vi "Teardown.vi"(8 "error in (no error)":errorcluster, 11 "Test Case Test Double In":refnum<class "Test Case Test Double.lvclass">) -> (0 "error out":errorcluster, 3 "Test Case Test Double Out":refnum<class "Test Case Test Double.lvclass">)   [LabVIEW 2020, in "Test Case Test Double.lvclass"]
uses:
  Test Case Test Double.lvclass
  source/Framework/Test Case/LUnit Test Case.lvclass
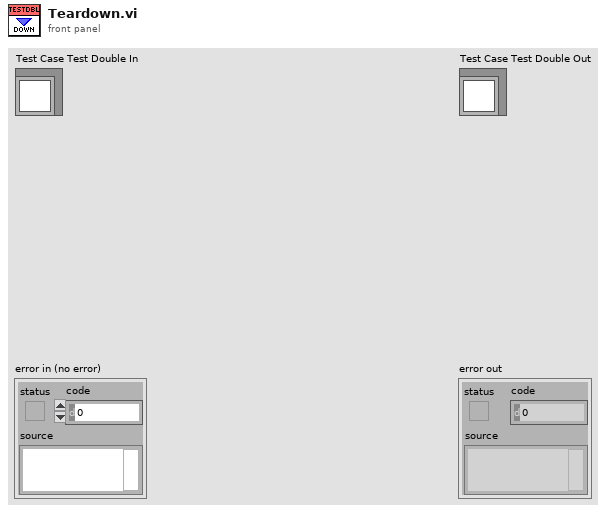
[diagram p1: front panel]
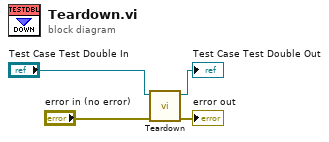
[diagram p0: block diagram]
diagram:
  n1 = call-parent "Teardown.vi"("error in (no error)"="error in (no error)", "LUnit Test Case In"="Test Case Test Double In") -> ("error out"=→"error out":errorcluster, "LUnit Test Case Out"=→"Test Case Test Double Out":refnum<class "Test Case Test Double.lvclass">)  [unwired: 8 in]
